vi "Write Ramp Volt.vi"(8 "error in":errorcluster, 10 "Voltage_Ramp":dbl, 11 "57XX in":refnum<class "57XX.lvclass">) -> (0 "error out":errorcluster, 3 "57XX out":refnum<class "57XX.lvclass">)   [LabVIEW 2019, in "57XX.lvlib" / "57XX.lvclass"]
uses:
  Library/57XX.lvclass
  C:/Users/Public/Documents/Development/builds/Engine/Monitored Actor.lvlibp/Monitored Actor/Monitored Actor/Monitored Actor.lvclass
  builds/Engine/Monitored Actor.lvlibp/Monitored Actor/Monitored Actor/Read Actor Label.vi
  builds/Instruments/PowerSupply.lvlibp/Library/PowerSupply.lvclass
  <vilib>/ErrorRing/Error Ring.xnode
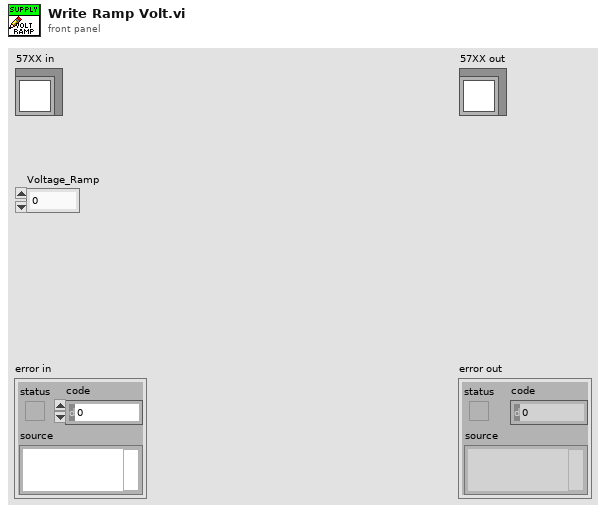
[diagram p1: front panel]
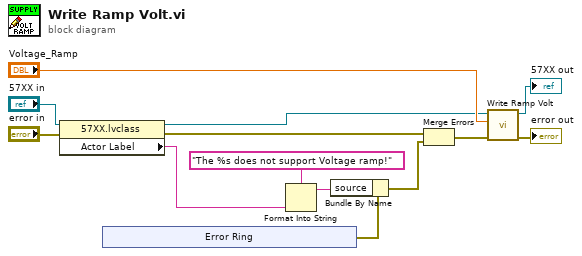
[diagram p0: block diagram]
diagram:
  n1 = property class="57XX.lvclass"(reference="57XX in", error in="error in") -> (reference out=w2:refnum<class "57XX.lvclass">, error out=w5:errorcluster, "Actor Label"=w9:string)
  n2 = xnode "Error Ring"() -> ("error out"=w6:errorcluster)
  n3 = Format Into String(format string="The %s does not support Voltage ramp!", w9) -> (resulting string=w7:string)  [unwired: 2 in, 1 out]
  n4 = Bundle By Name(cluster=w6, "source"=w7) -> (w8:errorcluster)
  n5 = Merge Errors(w5, w8) -> (w1:errorcluster)
  n6 = call-parent "Write Ramp Volt.vi"("error in"=w1, "Voltage_Ramp"="Voltage_Ramp", "PowerSupply in"=w2) -> ("error out"=→"error out":errorcluster, "PowerSupply out"=→"57XX out":refnum<class "57XX.lvclass">)  [unwired: 7 in]
